vi "SpeedAccelDeccelPositionM1M2.vi"(0 "VISA Refnum in":refnum<visa-resource-name>, 1 "Accel1":u32 max=127 step=1, 2 "Speed1":u32 max=127 step=1, 3 "Deccel1":u32 max=127 step=1, 5 "Address":u8, 8 "Position1":i32 max=127 step=1, 9 "Immediate":u8 max=127 step=1, 10 "Accel2":u32 max=127 step=1, 11 "error in (no error)":errorcluster, 12 "Position2":i32 max=127 step=1, 13 "Deccel2":u32 max=127 step=1, 14 "Speed2":u32 max=127 step=1) -> (4 "VISA Refnum out":refnum<visa-resource-name>, 6 "Valid":bool, 15 "error out":errorcluster)   [LabVIEW 2015, in "Ion Motion Roboclaw.lvlib"]
uses:
  <instrlib>/Ion Motion Roboclaw/Ion Motion Roboclaw.lvlib
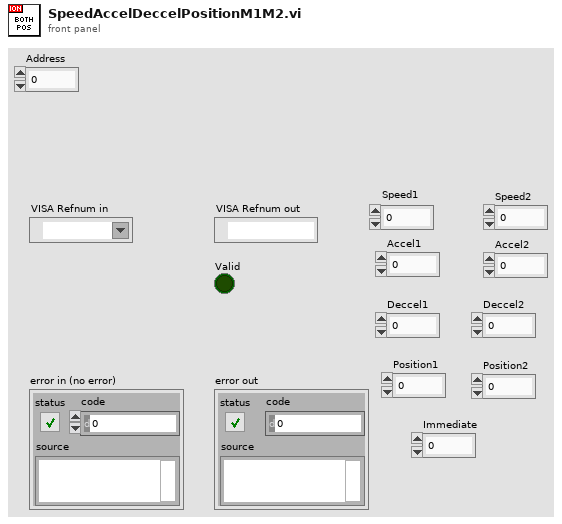
[diagram p1: front panel]
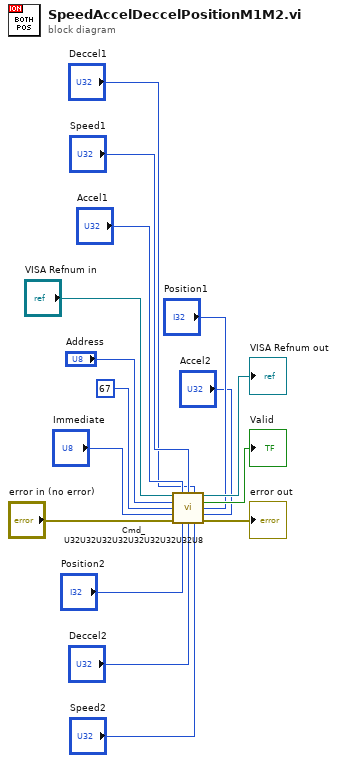
[diagram p0: block diagram]
diagram:
  n1 = call <instrlib>:"Cmd_U32U32U32U32U32U32U32U32U8.vi"("VISA Refnum in"="VISA Refnum in", "Arg1"="Accel1", "Arg2"="Speed1", "Arg3"="Deccel1", "Address"="Address", "Cmd"=u8 67, "Arg4"="Position1", "Arg9"="Immediate", "Arg5"="Accel2", "error in (no error)"="error in (no error)", "Arg8"="Position2", "Arg7"="Deccel2", "Arg6"="Speed2") -> ("VISA Refnum out"=→"VISA Refnum out":refnum<visa-resource-name>, "Valid"=→"Valid":bool, "error out"=→"error out":errorcluster)
